vi "dB to Linear (1D).vi"(1 "dB":dbl[](array[numeric])) -> (0 "linear":dbl[](array[numeric]))   [LabVIEW 2020]
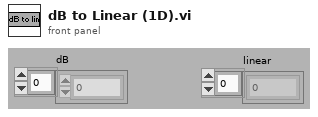
[diagram p1: front panel]
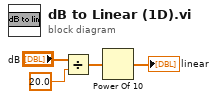
[diagram p0: block diagram]
diagram:
  n1 = Divide(x="dB", y=20.0) -> (x/y=w2:dbl[])
  n2 = Power Of 10(x=w2) -> (10^x=→"linear":dbl[])
